vi "Catalytic Methanation #2.vi"() -> ()   [LabVIEW 2017]
uses:
  <vilib>/addons/control/pid/pid.llb/PID Advanced (DBL).vi
  <vilib>/addons/control/pid/NI_PID_pid.lvlib
panel:
  out "Heater Temperature (C)":dbl format="%.2f"
  out "Last Time Write":dbl
  out "error constant":errorcluster
  out "Inlet Valve":bool
  in  "Replace File":bool
  in  "Recording Increment (sec)":dbl=0.3 min=0.1 max=100.0 step=0.1 format="%#_13g"
  in  "Record":bool
  out "Heater On?":bool
  in  "Heater Switch":bool
  in  "CO2 Setpoint (SCCM)":dbl min=0.0 max=10.0 format="%.2f"
  in  "Temperature Setpoint (C)":dbl=20.0 min=0.0 max=325.0 format="%.1f"
  out "Reactor Temperature (C)":dbl format="%.2f"
  out "Heater Output (%)":dbl(slide) scale=0.0..100.0
  in  "Manual Control Override (Temperature)":bool=TRUE
  in  "Set Manual Valve Heater Output (Temperature)":dbl(slide) scale=0.0..100.0
  in  "Reactor Pressure  Setpoint (psia)":dbl=18.4 min=0.0 max=30.0 format="%.1f"
  out "Reactor Pressure (psia)":dbl format="%.1f"
  out "Pressure Control Valve (%)":dbl(slide) scale=0.0..100.0
  in  "Manual Control Override (Pressure)":bool=TRUE
  in  "Set Manual Valve Position (Pressure)":dbl(slide)=50.0 scale=0.0..100.0
  in  "stop":bool
  in  "H2 Setpoint (SCCM)":dbl min=0.0 max=50.0 format="%.2f"
  in  "He Setpoint (SCCM)":dbl min=0.0 max=200.0 format="%.1f"
  out "CO2 Flowrate (SCCM)":dbl format="%.2f"
  out "H2 Flowrate (SCCM)":dbl format="%.2f"
  out "He Flowrate (SCCM)":dbl format="%.1f"
  in  "GC Sample Path":enum32{"Reactor Feed", "Reactor Exhaust"}(radio)=enum."Reactor Exhaust"
  in  "Kc (Heater)":dbl=3.0
  in  "Ti (Heater)":dbl=5.0 caption="(min)"
  in  "Td (Heater)":dbl caption="(min)"
  in  "Kc (Pressure)":dbl=-0.1
  in  "Ti (Pressure)":dbl=0.01
  in  "Td (Pressure)":dbl
  # "Heater Power"
  # "Total Flow > 190 SCCM\nH2/CO2 > 3.85\nGC Sample Path: Reactor Exhaust"
  # "Gas Flow Rates (SCCM)"
  # "Setpoint"
  # "Actual"
  # "Hydrogen"
  # "Carbon Dioxide"
  # "Helium"
  # "Data Collection"
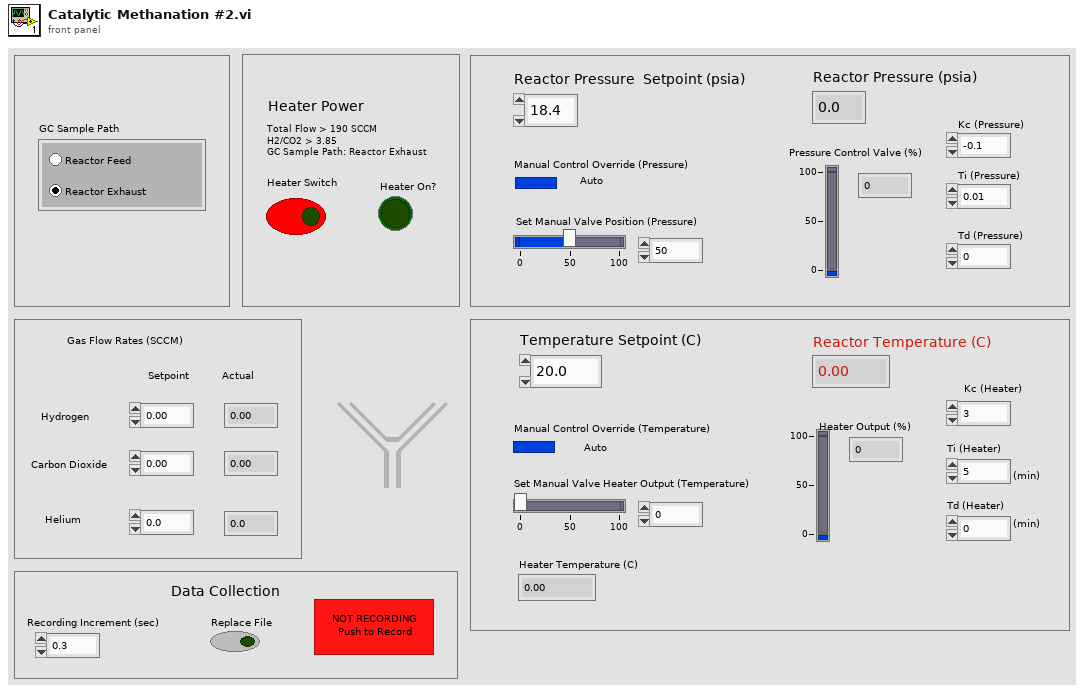
[diagram p1: front panel]
types:
  T1 = enum16{"open", "replace", "create", "open or create", "replace or create", "replace or create with confirmation"}
  T2 = cluster{"Kc (Heater)":dbl, "Ti (Heater)":dbl, "Td (Heater)":dbl}
  T3 = cluster{"Kc (Pressure)":dbl, "Ti (Pressure)":dbl, "Td (Pressure)":dbl}
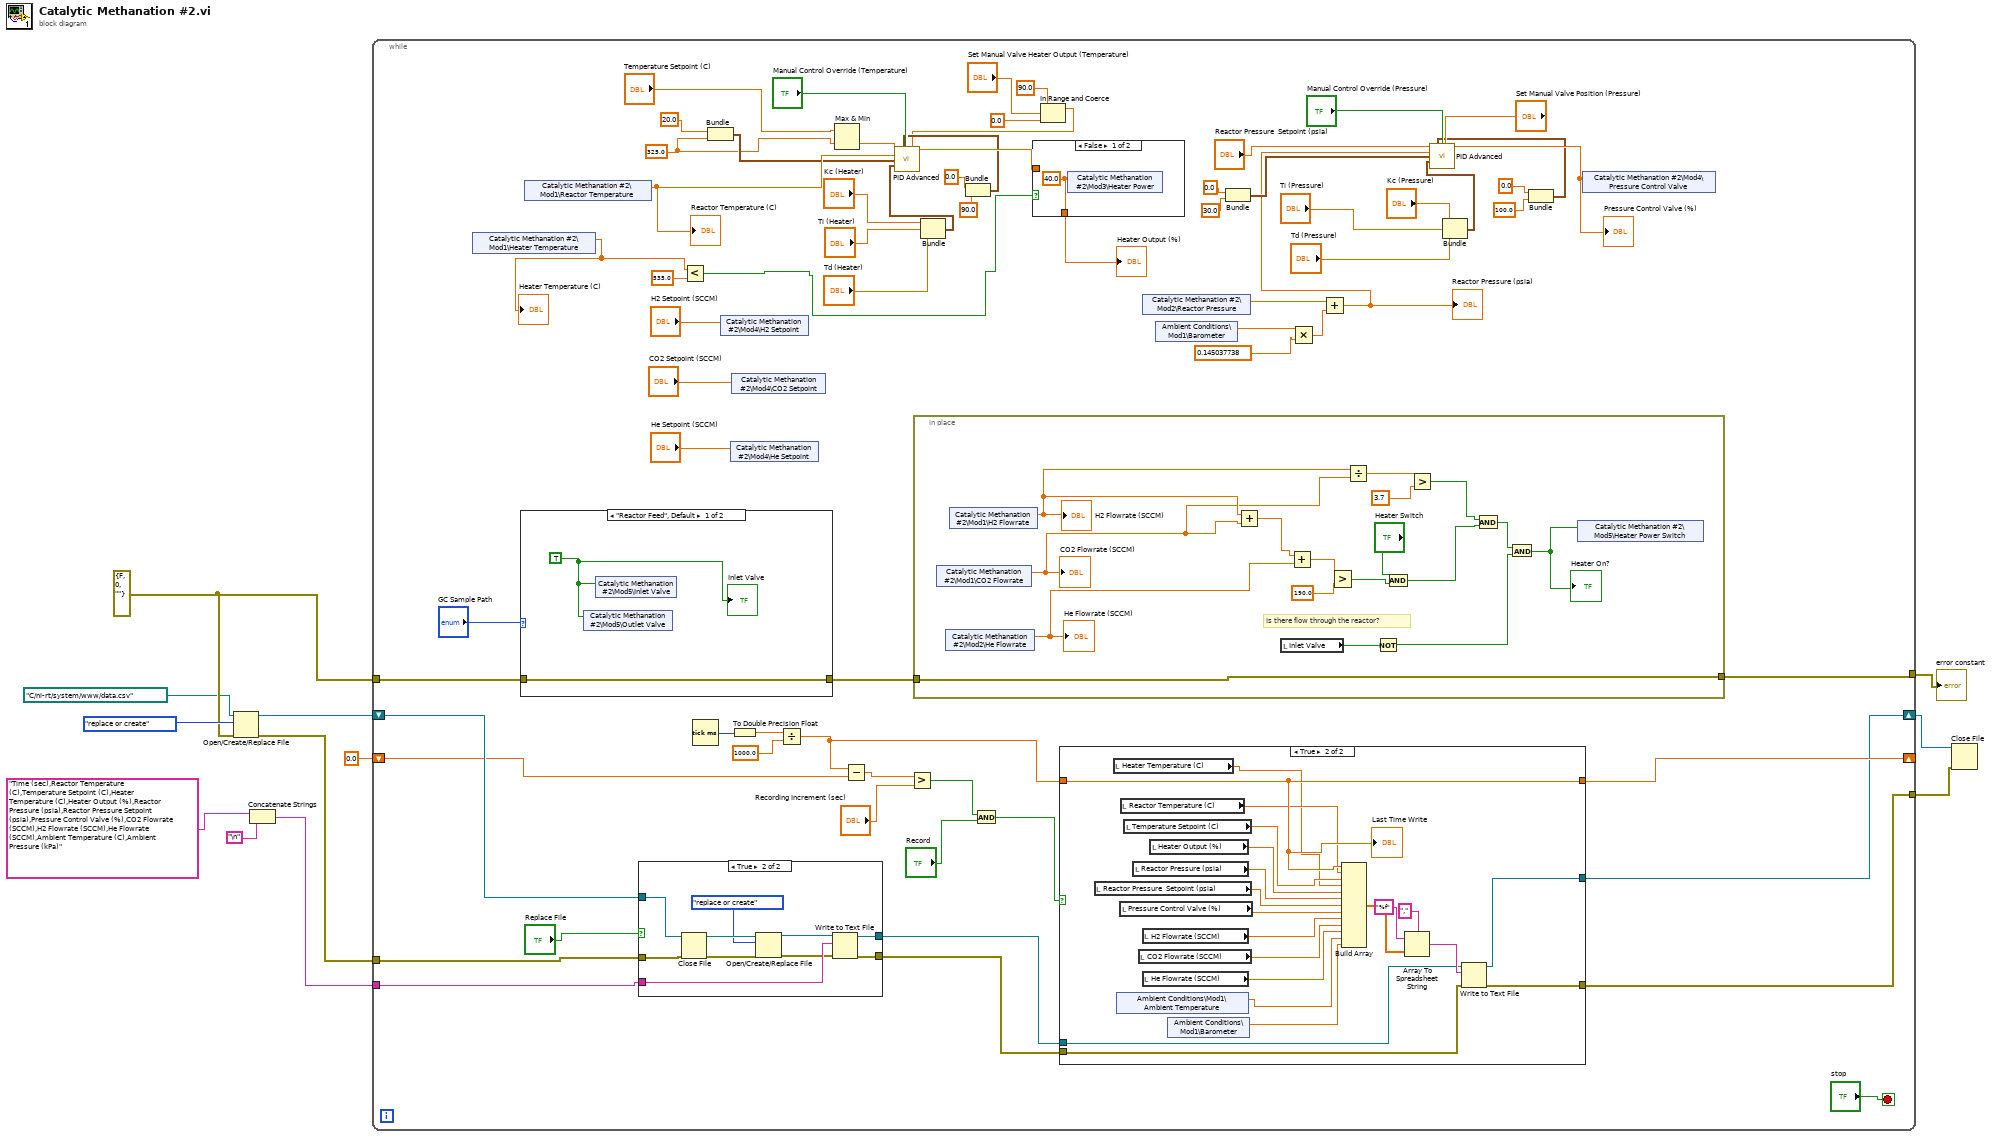
[diagram p0: block diagram]
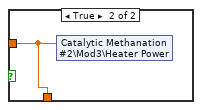
[diagram p2: hidden frame]
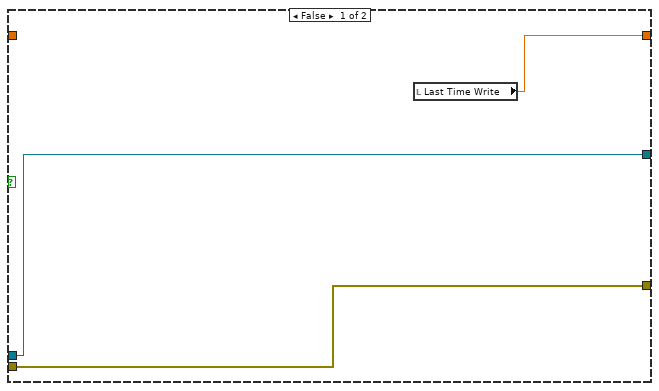
[diagram p3: hidden frame]
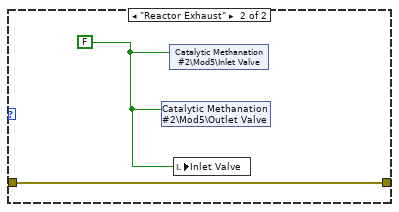
[diagram p5: hidden frame]
diagram:
  w9 = errorcluster {"status"=FALSE, "code"=0, "source"=""} ("error constant")
  n1 = Open/Create/Replace File(file path (use dialog)=path "C:/ni-rt/system/www/data.csv" ("Filename"), error in=w9, operation (0:open)=T1."replace or create") -> (refnum out=w7:refnum<file>, error out=w6:errorcluster)  [unwired: 3 in, 1 out]
  n2 = Concatenate Strings("Time (sec),Reactor Temperature (C),Temperature Setpoint (C),Heater Temperature (C),Heater Output (%),Reactor Pressure (psia),Reactor Pressure Setpoint (psia),Pressure Control Valve (%),CO2 Flowrate (SCCM),H2 Flowrate (SCCM),He Flowrate (SCCM),Ambient Temperature (C),Ambient Pressure (kPa)", "\n") -> (w5:string)
  n3 = while {
    tunnel: w9 -> [w38]
    shift-right: [w18] -> w2
    shift-left: w7 -> [w36]
    tunnel: w6 -> [w35]
    tunnel: w5 -> [w34]
    shift-right: [w19] -> _
    shift-left: 0.0 ("Last Time Write") -> [w30]
    tunnel: [w25] -> w3
    tunnel: [w17] -> w1
    stop <- "stop" stop-if-true
    w58 = 325.0
    n4 = shared-variable "Catalytic Methanation #2\\Mod1\\Heater Temperature"() -> (w15:dbl)  [unwired: 1 in, 1 out]
    "Heater Temperature (C)" <- w15
    n5 = case shown="\"Reactor Feed\", Default" "GC Sample Path" {
      tunnel: [w137 w139] -> w24
      tunnel: w38 -> [w137 w139]
      frame "Reactor Feed", Default {
        w138 = TRUE ("Inlet Valve")
        n6 = shared-variable "Catalytic Methanation #2\\Mod5\\Outlet Valve"(w138) -> ()  [unwired: 1 in, 1 out]
        n7 = shared-variable "Catalytic Methanation #2\\Mod5\\Inlet Valve"(w138) -> ()  [unwired: 1 in, 1 out]
        "Inlet Valve" <- w138
      }
      frame "Reactor Exhaust" {
        w140 = FALSE ("Inlet Valve")
        n8 = shared-variable "Catalytic Methanation #2\\Mod5\\Outlet Valve"(w140) -> ()  [unwired: 1 in, 1 out]
        n9 = shared-variable "Catalytic Methanation #2\\Mod5\\Inlet Valve"(w140) -> ()  [unwired: 1 in, 1 out]
        n10 = local write "Inlet Valve"(w140) -> ()
      }
    }
    n11 = shared-variable "Catalytic Methanation #2\\Mod1\\Reactor Temperature"() -> (w68:dbl)  [unwired: 1 in, 1 out]
    "Reactor Temperature (C)" <- w68
    n12 = case shown="True" "Replace File" {
      tunnel: w34 -> [_ w134]
      tunnel: w36 -> [w126 w132]
      tunnel: [w126 w131] -> w21
      tunnel: w35 -> [w125 w130]
      tunnel: [w125 w127] -> w20
      frame False {
      }
      frame True {
        n13 = Close File(refnum=w132, error in=w130) -> (path=w135:path, error out=w129:errorcluster)
        n14 = Open/Create/Replace File(file path (use dialog)=w135, error in=w129, operation (0:open)=T1."replace or create") -> (refnum out=w136:refnum<file>, error out=w128:errorcluster)  [unwired: 3 in, 1 out]
        n15 = Write to Text File(file (use dialog)=w136, text=w134, error in=w128) -> (refnum out=w131:refnum<file>, error out=w127:errorcluster)  [unwired: 1 in, 1 out]
      }
    }
    n16 = Less?(x=w15, y=535.0) -> (x < y?=w14:bool)
    n17 = Tick Count (ms)() -> (millisecond timer value=w33:u32)
    n18 = Bundle(20.0, w58) -> (w60:cluster{dbl, dbl})  [unwired: 1 in]
    n19 = shared-variable "Catalytic Methanation #2\\Mod4\\H2 Setpoint"("H2 Setpoint (SCCM)") -> ()  [unwired: 1 in, 1 out]
    n20 = shared-variable "Catalytic Methanation #2\\Mod4\\He Setpoint"("He Setpoint (SCCM)") -> ()  [unwired: 1 in, 1 out]
    n21 = shared-variable "Catalytic Methanation #2\\Mod4\\CO2 Setpoint"("CO2 Setpoint (SCCM)") -> ()  [unwired: 1 in, 1 out]
    n22 = To Double Precision Float(number=w33) -> (double precision float=w32:dbl)
    n23 = Divide(x=w32, y=1000.0) -> (x/y=w22:dbl)
    n24 = Max & Min(x="Temperature Setpoint (C)", y=w58) -> (min(x,y)=w50:dbl)  [unwired: 1 out]
    n25 = Subtract(x=w22, y=w30) -> (x-y=w27:dbl)
    n26 = Greater?(x=w27, y="Recording Increment (sec)") -> (0:w29:bool)
    n27 = in-place {
      in-place-border: [w108] -> w25
      in-place-border: w24 -> [w108]
      # "Is there flow through the reactor?"
      n28 = shared-variable "Catalytic Methanation #2\\Mod1\\CO2 Flowrate"() -> (w117:dbl)  [unwired: 1 in, 1 out]
      "CO2 Flowrate (SCCM)" <- w117
      n29 = shared-variable "Catalytic Methanation #2\\Mod2\\He Flowrate"() -> (w123:dbl)  [unwired: 1 in, 1 out]
      "He Flowrate (SCCM)" <- w123
      n30 = shared-variable "Catalytic Methanation #2\\Mod1\\H2 Flowrate"() -> (w118:dbl)  [unwired: 1 in, 1 out]
      "H2 Flowrate (SCCM)" <- w118
      n31 = Add(x=w118, y=w117) -> (x+y=w124:dbl)
      n32 = local read "Inlet Valve"() -> (w112:bool)
      n33 = Add(x=w124, y=w123) -> (x+y=w122:dbl)
      n34 = Greater?(x=w122, y=190.0) -> (0:w119:bool)
      n35 = Divide(x=w118, y=w117) -> (x/y=w116:dbl)
      n36 = Not(x=w112) -> (.not. x?=w109:bool)
      n37 = And(x="Heater Switch", y=w119) -> (x .and. y?=w113:bool)
      n38 = Greater?(x=w116, y=3.7) -> (0:w114:bool)
      n39 = And(x=w114, y=w113) -> (x .and. y?=w110:bool)
      n40 = And(x=w110, y=w109) -> (x .and. y?=w111:bool)
      "Heater On?" <- w111
      n41 = shared-variable "Catalytic Methanation #2\\Mod5\\Heater Power Switch"(w111) -> ()  [unwired: 1 in, 1 out]
    }
    n42 = Bundle("Kc (Heater)"="Kc (Heater)", "Ti (Heater)"="Ti (Heater)", "Td (Heater)"="Td (Heater)") -> (w77:T2)  [unwired: 1 in]
    n43 = Bundle(0.0, 90.0) -> (w62:cluster{dbl, dbl})  [unwired: 1 in]
    n44 = And(x=w29, y="Record") -> (x .and. y?=w23:bool)
    n45 = In Range and Coerce(upper limit=90.0, x="Set Manual Valve Heater Output (Temperature)", lower limit=0.0) -> (coerced(x)=w48:dbl)  [unwired: 1 out]
    n46 = call-poly <vilib>:"PID Advanced.vi"("setpoint"=w50, "output range"=w62, "auto? (T)"="Manual Control Override (Temperature)", "manual control"=w48, "process variable"=w68, "setpoint range"=w60, "PID gains"=w77) -> ("output"=w70:dbl)  [unwired: 7 in, 1 out]
    n47 = case shown="False" w14 {
      tunnel: w70 -> [_ w83]
      tunnel: [w82 w83] -> w13
      frame False {
        w82 = 40.0 ("Heater Power")
        n48 = shared-variable "Catalytic Methanation #2\\Mod3\\Heater Power"(w82) -> ()  [unwired: 1 in, 1 out]
      }
      frame True {
        n49 = shared-variable "Catalytic Methanation #2\\Mod3\\Heater Power"(w83) -> ()  [unwired: 1 in, 1 out]
      }
    }
    "Heater Output (%)" <- w13
    n50 = case shown="True" w23 {
      tunnel: w22 -> [_ w90]
      tunnel: [w86 w90] -> w19
      tunnel: w21 -> [w85 w94]
      tunnel: w20 -> [w84 w93]
      tunnel: [w85 w92] -> w18
      tunnel: [w84 w91] -> w17
      frame False {
        n51 = local read "Last Time Write"() -> (w86:dbl)
      }
      frame True {
        n52 = local read "Reactor Pressure  Setpoint (psia)"() -> (w97:dbl)
        n53 = local read "Heater Temperature (C)"() -> (w87:dbl)
        n54 = shared-variable "Ambient Conditions\\Mod1\\Ambient Temperature"() -> (w102:dbl)  [unwired: 1 in, 1 out]
        n55 = local read "Pressure Control Valve (%)"() -> (w98:dbl)
        n56 = local read "Reactor Temperature (C)"() -> (w89:dbl)
        n57 = local read "Temperature Setpoint (C)"() -> (w88:dbl)
        n58 = local read "Reactor Pressure (psia)"() -> (w96:dbl)
        n59 = local read "CO2 Flowrate (SCCM)"() -> (w100:dbl)
        n60 = local read "H2 Flowrate (SCCM)"() -> (w99:dbl)
        n61 = local read "He Flowrate (SCCM)"() -> (w101:dbl)
        n62 = local read "Heater Output (%)"() -> (w95:dbl)
        n63 = shared-variable "Ambient Conditions\\Mod1\\Barometer"() -> (w103:dbl)  [unwired: 1 in, 1 out]
        n64 = Build Array(w90, w89, w88, w87, w95, w96, w97, w98, w99, w100, w101, w102, w103) -> (w107:dbl[])
        n65 = Array To Spreadsheet String(delimiter (Tab)=",", array=w107, 3:"%f") -> (spreadsheet string=w104:string)
        n66 = Write to Text File(file (use dialog)=w94, text=w104, error in=w93) -> (refnum out=w92:refnum<file>, error out=w91:errorcluster)  [unwired: 1 in, 1 out]
        "Last Time Write" <- w90
      }
    }
    n67 = shared-variable "Catalytic Methanation #2\\Mod2\\Reactor Pressure"() -> (w40:dbl)  [unwired: 1 in, 1 out]
    n68 = shared-variable "Ambient Conditions\\Mod1\\Barometer"() -> (w44:dbl)  [unwired: 1 in, 1 out]
    n69 = Bundle(0.0, 30.0) -> (w56:cluster{dbl, dbl})  [unwired: 1 in]
    n70 = Multiply(x=w44, y=0.145037738) -> (x*y=w42:dbl)
    n71 = Add(x=w40, y=w42) -> (x+y=w41:dbl)
    "Reactor Pressure (psia)" <- w41
    n72 = Bundle("Kc (Pressure)"="Kc (Pressure)", "Ti (Pressure)"="Ti (Pressure)", "Td (Pressure)"="Td (Pressure)") -> (w78:T3)  [unwired: 1 in]
    n73 = Bundle(0.0, 100.0) -> (w53:cluster{dbl, dbl})  [unwired: 1 in]
    n74 = call-poly <vilib>:"PID Advanced.vi"("setpoint"="Reactor Pressure  Setpoint (psia)", "output range"=w53, "auto? (T)"="Manual Control Override (Pressure)", "manual control"="Set Manual Valve Position (Pressure)", "process variable"=w41, "setpoint range"=w56, "PID gains"=w78) -> ("output"=w81:dbl)  [unwired: 7 in, 1 out]
    "Pressure Control Valve (%)" <- w81
    n75 = shared-variable "Catalytic Methanation #2\\Mod4\\Pressure Control Valve"(w81) -> ()  [unwired: 1 in, 1 out]
  }
  "error constant" <- w3
  n76 = Close File(refnum=w2, error in=w1) -> ()  [unwired: 2 out]
